vi "test_Corner and Feature Point Detection.vi"() -> ()   [LabVIEW 2020]
doc: "This example illustrates Harris, Shi-Tomasi corner detection and FAST feature point detection algorithms. Part image is calibrated to correct the distortions and flat field correction is used to correct the non-uniform intensity. Corner and feature points are detected in real world units and circle fit is used to find the radius of the object."
uses:
  <vilib>/vision/NI_Vision_Development_Module.lvlib
panel:
  in  "Tab Control":enum32{"Part Images", "Templates"}(tab)
  out "Processed Part Image":T1(plugin-control)
  out "Part Image":T1(plugin-control)
  out "Flat Field Image":T1(plugin-control)
  out "Calibration Template":T1(plugin-control)
  in  "Detector Type":enum16{"FAST", "Harris", "Shi-Tomasi"}(ring)
  in  "Stop":bool
  in  "Select Image":i32(slide) min=0 max=5 step=1 scale=0.0..4.0
  # "Overview: Demonstrates how to detect real world feature points using IMAQ FAST Feature Point Detector and IMAQ Corner Detector and how to correct non-uniform intensity before proceeding to feature point detection.\nInstructions:\n1. Run the VI.\n2. Choose images using Select Image control.\n3. Choose detector using Detector Type\n3. Observe the feature points overlay in Processed Image control\n4. Observe that radius (in cm) of the object is calculated using real world feature points and circle fit."
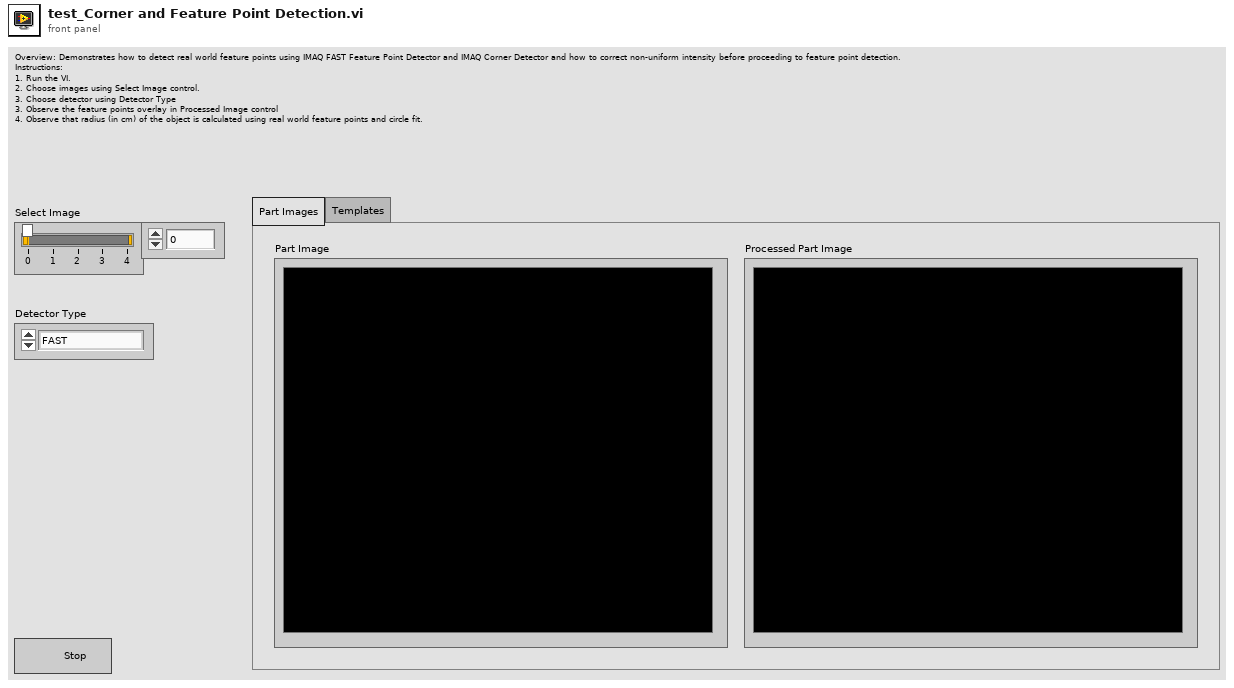
[diagram p1: front panel]
types:
  T1 = typedef "IMAQ Image.ctl" = refnum<image>
  T2 = cluster{"Line Scan Image?":bool, "Correction Factor":sgl}
  T3 = cluster{"Detector type":enum32{"Harris Corner", "Shi-Tomasi Corner"}, "Kernel size":i32, "Min Corner Point Strength":dbl}
  T4 = cluster{"Center":cluster{"X":sgl, "Y":sgl}, "Radius":dbl}
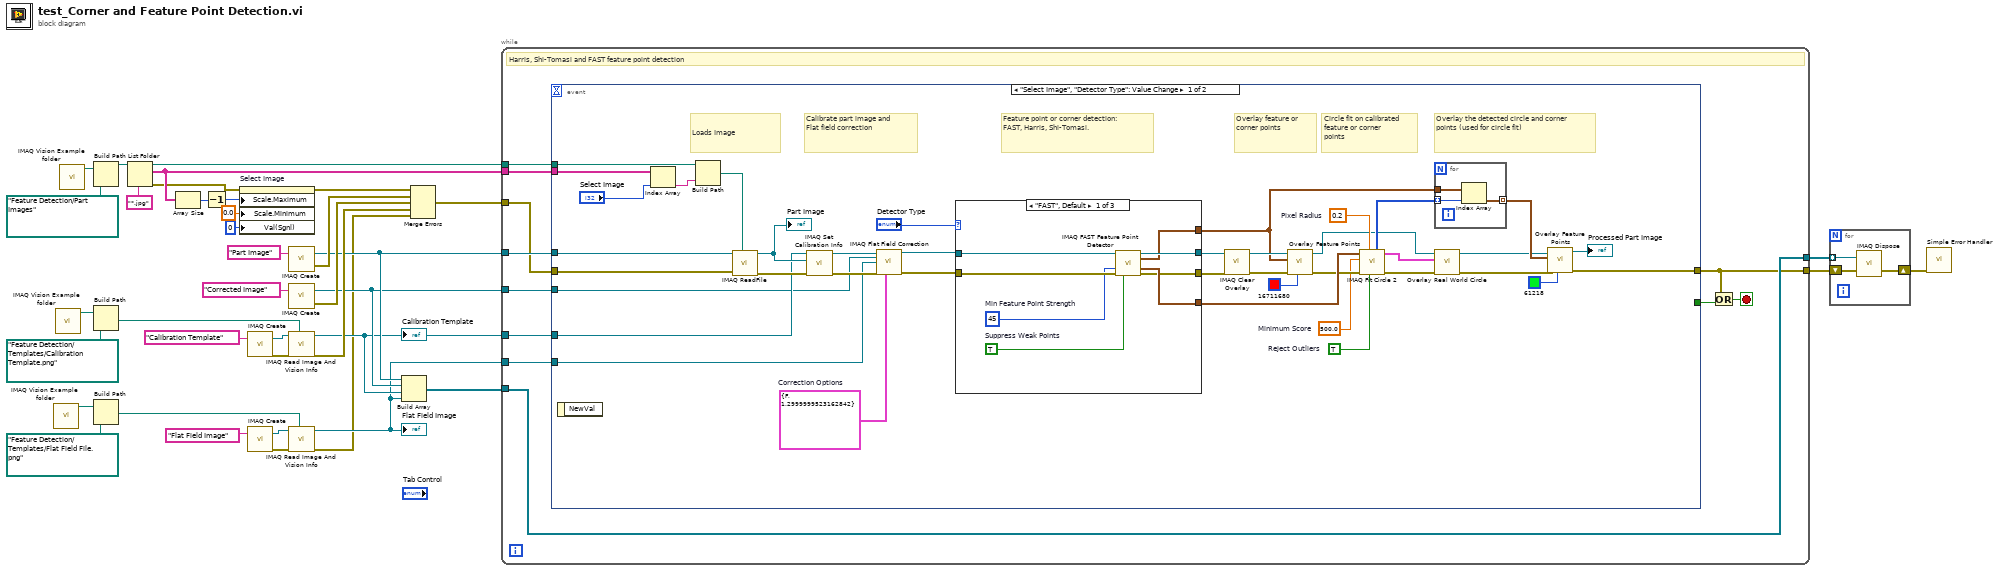
[diagram p0: block diagram]
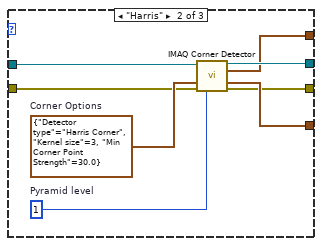
[diagram p2: hidden frame]
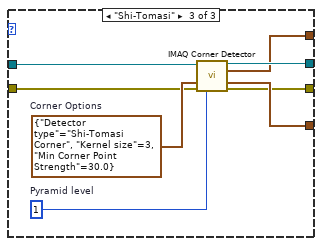
[diagram p3: hidden frame]
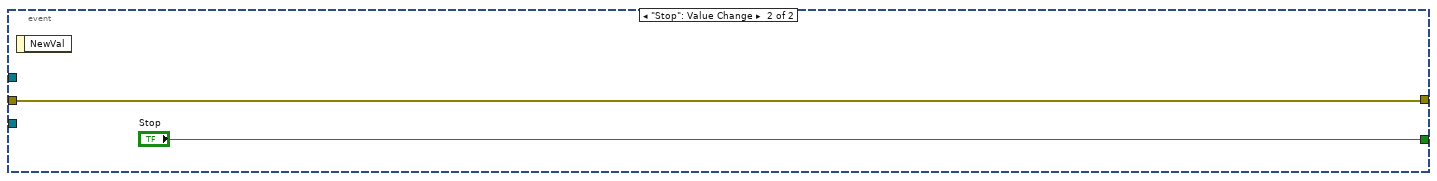
[diagram p4: hidden frame]
diagram:
  n1 = call "IMAQ Vision Example folder.vi"() -> ("Example Image Path"=w11:path)  [unwired: 11 in]
  n2 = call "IMAQ Vision Example folder.vi"() -> ("Example Image Path"=w10:path)  [unwired: 11 in]
  n3 = call "IMAQ Vision Example folder.vi"() -> ("Example Image Path"=w9:path)  [unwired: 11 in]
  n4 = Build Path(base path=w9, name or relative path=path "Feature Detection/Part Images" ("appended path")) -> (appended path=w37:path)
  n5 = Build Path(base path=w10, name or relative path=path "Feature Detection/Templates/Calibration Template.png" ("appended path")) -> (appended path=w19:path)
  n6 = Build Path(base path=w11, name or relative path=path "Feature Detection/Templates/Flat Field File.png" ("appended path")) -> (appended path=w15:path)
  n7 = List Folder(path=w37, pattern="*.jpg") -> (path out=w38:path, filenames=w39:string[], error out=w26:errorcluster)  [unwired: 1 in, 2 out]
  n8 = Array Size(array=w39) -> (size(s)=w33:i32)
  n9 = Decrement(x=w33) -> (x-1=w32:i32)
  n10 = property on="Select Image" class="Slide (strict)"(error in=w26, "Scale.Maximum"=w32, "Scale.Minimum"=0.0 ("Scale.Range:Minimum"), "Val(Sgnl)"=0 ("Value (Signaling)")) -> (error out=w25:errorcluster)  [unwired: 1 in, 1 out]
  n11 = call "IMAQ Create"("Image Name"="Calibration Template") -> ("New Image"=w20:T1, "error out"=w21:errorcluster)  [unwired: 4 in]
  n12 = call "IMAQ Create"("Image Name"="Flat Field Image") -> ("New Image"=w18:T1, "error out"=w17:errorcluster)  [unwired: 4 in]
  n13 = call "IMAQ Create"("Image Name"="Part Image") -> ("New Image"=w5:T1, "error out"=w28:errorcluster)  [unwired: 4 in]
  n14 = call "IMAQ Create"("Image Name"="Corrected Image") -> ("New Image"=w4:T1, "error out"=w6:errorcluster)  [unwired: 4 in]
  n15 = call "IMAQ Read Image And Vision Info"("File Path"=w19, "error in (no error)"=w21, "Image"=w20) -> ("error out"=w7:errorcluster, "Image Out"=w3:T1)  [unwired: 6 in, 1 out]
  "Calibration Template" <- w3
  n16 = call "IMAQ Read Image And Vision Info"("File Path"=w15, "error in (no error)"=w17, "Image"=w18) -> ("error out"=w1:errorcluster, "Image Out"=w2:T1)  [unwired: 6 in, 1 out]
  "Flat Field Image" <- w2
  n17 = Build Array(w5, w4, w3, w2) -> (w13:T1[])
  n18 = Merge Errors(w25, w28, w6, w7, w1) -> (w24:errorcluster)
  n19 = while {
    tunnel: w39 -> [w50]
    tunnel: w38 -> [w49]
    tunnel: w5 -> [w48]
    tunnel: w24 -> [w47]
    tunnel: w3 -> [w46]
    tunnel: w2 -> [w45]
    tunnel: [w41] -> w14
    tunnel: w13 -> [w44]
    tunnel: [w44] -> w12
    tunnel: w4 -> [w43]
    stop <- w40 stop-if-true
    # "Harris, Shi-Tomasi and FAST feature point detection"
    n20 = event shown="[0] \"Select Image\", \"Detector Type\": Value Change" {
      selector: _ -> [_ _]
      dyn-events: _ -> [_ _]
      timeout: _ -> [_ _]
      tunnel: w48 -> [w85 _]
      tunnel: w46 -> [w64 _]
      tunnel: w45 -> [w65 _]
      tunnel: w49 -> [w89 _]
      tunnel: w50 -> [w88 _]
      tunnel: w47 -> [w82 w117]
      tunnel: [w55 w117] -> w41
      tunnel: [_ "Stop"] -> w42
      tunnel: w43 -> [w51 _]
      event "Select Image", "Detector Type": Value Change {
        w61 = 500.0  # Minimum Score
        w62 = 0.2  # Pixel Radius
        w63 = TRUE  # Reject Outliers
        w68 = T2 {"Line Scan Image?"=FALSE, "Correction Factor"=1.3}  # Correction Options
        # "Overlay feature or corner points"
        # "Overlay the detected circle and corner points (used for circle fit)"
        # "Circle fit on calibrated feature or corner points"
        # "Feature point or corner detection: FAST, Harris, Shi-Tomasi."
        # "Calibrate part image and\nFlat field correction"
        # "Loads Image"
        n21 = event-data() -> ()  [unwired: 1 in, 1 out]
        n22 = Index Array(array=w88, index="Select Image") -> (element=w86:string)
        n23 = Build Path(base path=w89, name or relative path=w86) -> (appended path=w84:path)
        n24 = call "IMAQ ReadFile"("File Path"=w84, "error in (no error)"=w82, "Image"=w85) -> ("error out"=w81:errorcluster, "Image Out"=w83:T1)  [unwired: 4 in, 3 out]
        "Part Image" <- w83
        n25 = call "IMAQ Set Calibration Info"("error in (no error)"=w81, "Image Dst"=w83, "Image Src"=w64) -> ("error out"=w71:errorcluster, "Calibrated Image"=w72:T1)  [unwired: 7 in]
        n26 = call "IMAQ Flat Field Correction"("Image Src"=w72, "Image Dst"=w51, "Flat Field Image"=w65, "error in (no error)"=w71, "Correction Options"=w68) -> ("Corrected Image"=w69:T1, "error out"=w70:errorcluster)  [unwired: 8 in, 1 out]
        n27 = case shown="\"FAST\", Default" "Detector Type" {
          tunnel: w69 -> [w99 w105 w113]
          tunnel: w70 -> [w100 w106 w114]
          tunnel: [w96 w104 w112] -> w74
          tunnel: [w95 w103 w111] -> w79
          tunnel: [w94 w102 w110] -> w78
          tunnel: [w93 w101 w109] -> w59
          frame "FAST", Default {
            w97 = 45  # Min Feature Point Strength
            w98 = TRUE  # Suppress Weak Points
            n28 = call "IMAQ FAST Feature Point Detector"("Image"=w99, "Min Feature Point Strength"=w97, "error in (no error)"=w100, "Suppress Weak Points"=w98) -> ("Image (duplicate)"=w95:T1, "Feature Point Coordinates"=w93:cluster{"X":sgl, "Y":sgl}[], "Feature Point Coordinates (Real)"=w96:cluster{"X":sgl, "Y":sgl}[], "error out"=w94:errorcluster)  [unwired: 6 in, 2 out]
          }
          frame "Harris" {
            w107 = u32 1  # Pyramid level
            w108 = T3 {"Detector type"=enum."Harris Corner", "Kernel size"=3, "Min Corner Point Strength"=30.0}  # Corner Options
            n29 = call "IMAQ Corner Detector"("Image"=w105, "Corner Options"=w108, "error in (no error)"=w106, "Pyramid level"=w107) -> ("Image (duplicate)"=w103:T1, "Corner Point Coordinates"=w101:cluster{"X":sgl, "Y":sgl}[], "Corner Point Coordinates (Real)"=w104:cluster{"X":sgl, "Y":sgl}[], "error out"=w102:errorcluster)  [unwired: 6 in, 2 out]
          }
          frame "Shi-Tomasi" {
            w115 = u32 1  # Pyramid level
            w116 = T3 {"Detector type"=enum."Shi-Tomasi Corner", "Kernel size"=3, "Min Corner Point Strength"=30.0}  # Corner Options
            n30 = call "IMAQ Corner Detector"("Image"=w113, "Corner Options"=w116, "error in (no error)"=w114, "Pyramid level"=w115) -> ("Image (duplicate)"=w111:T1, "Corner Point Coordinates"=w109:cluster{"X":sgl, "Y":sgl}[], "Corner Point Coordinates (Real)"=w112:cluster{"X":sgl, "Y":sgl}[], "error out"=w110:errorcluster)  [unwired: 6 in, 2 out]
          }
        }
        n31 = call "IMAQ Clear Overlay"("error in (no error)"=w78, "Image"=w79) -> ("error out"=w77:errorcluster, "Image Out"=w76:T1)  [unwired: 8 in]
        n32 = call "Overlay Feature Points.vi"("Color"=u32 16711680, "error in"=w77, "Feature Points"=w59, "Image"=w76) -> ("error out"=w73:errorcluster, "Image Out"=w52:T1)  [unwired: 6 in]
        n33 = call "IMAQ Fit Circle 2"("Reject Outliers (FALSE)"=w63, "Pixel Radius"=w62, "error in (no error)"=w73, "Minimum Score"=w61, "Radial Points"=w74) -> ("error out"=w54:errorcluster, "Circle"=w58:T4, "Indexes of Points Used"=w67:i32[])  [unwired: 1 in, 3 out]
        n34 = for {
          tunnel: w67 -> [w92] mode=indexing
          tunnel: w59 -> [w91]
          tunnel: [w90] -> w60 mode=indexing
          n35 = Index Array(array=w91, index=w92) -> (element=w90:cluster{"X":sgl, "Y":sgl})
        }
        n36 = call "Overlay Real World Circle.vi"("error in (no error)"=w54, "Circle (Real World)"=w58, "Image"=w52) -> ("error out"=w53:errorcluster, "Image Out"=w57:T1)  [unwired: 7 in]
        n37 = call "Overlay Feature Points.vi"("Color"=u32 61218, "error in"=w53, "Feature Points"=w60, "Image"=w57) -> ("error out"=w55:errorcluster, "Image Out"=→"Processed Part Image":T1)  [unwired: 6 in]
      }
      event "Stop": Value Change {
        n38 = event-data() -> ()  [unwired: 1 in, 1 out]
      }
    }
    n39 = Or(x=w41, y=w42) -> (x .or. y?=w40:bool)
  }
  n40 = for {
    shift-right: [w121] -> w27
    shift-left: w14 -> [w120]
    tunnel: w12 -> [w119] mode=indexing
    n41 = call "IMAQ Dispose"("Image"=w119, "error in (no error)"=w120) -> ("error out"=w121:errorcluster)  [unwired: 4 in]
  }
  n42 = call <vilib>:"Simple Error Handler.vi"("error in (no error)"=w27) -> ()  [unwired: 4 in, 5 out]
